vi "Initialise.vi"(8 "error in (no error)":errorcluster, 11 "Actor in":refnum<class "Status Window.lvclass">) -> (0 "error out":errorcluster, 3 "Actor out":refnum<class "Status Window.lvclass">, 5 "Observers":cluster{"Actor":refnum<event-registration>})   [LabVIEW 2015, in "Status Window.lvclass"]
uses:
  Status Window.lvclass
  Re-use Libraries/Minimal Actor Framework/Messaging/Message/Message.lvclass
  Re-use Libraries/Utility/Utility.lvlib
  Re-use Libraries/Minimal Actor Framework/Actors/Base Actor/Actor/Actor.lvclass
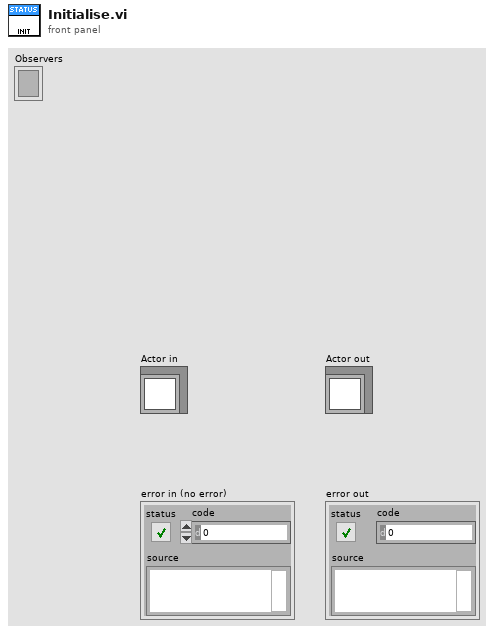
[diagram p1: front panel]
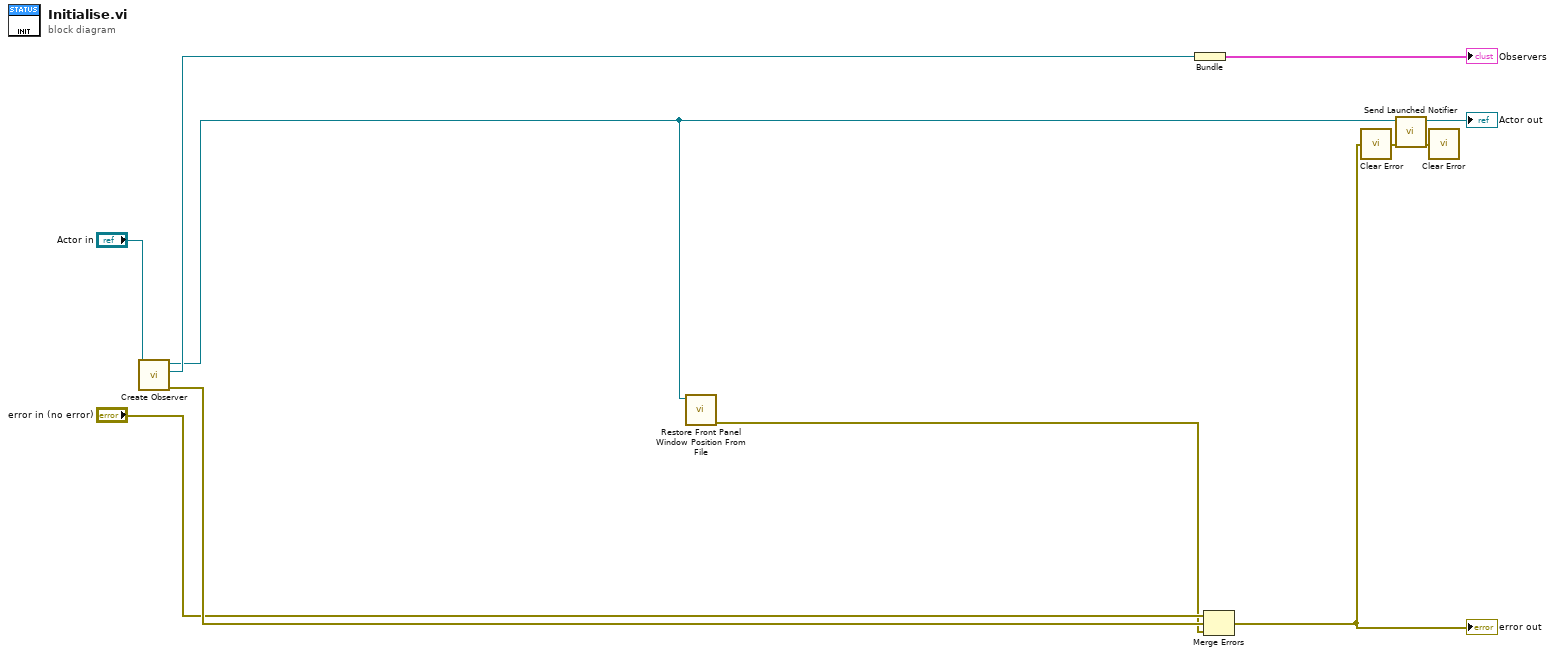
[diagram p0: block diagram]
diagram:
  n1 = call-dynamic "Create Observer.vi"("Actor in"="Actor in") -> ("error out"=w9:errorcluster, "Actor"=w4:refnum<event-registration>, "Actor out"=w1:refnum<class "Status Window.lvclass">)  [unwired: 8 in]
  n2 = call "Restore Front Panel Window Position From File.vi"("Actor in"=w1) -> ("error out"=w2:errorcluster)  [unwired: 10 in]
  n3 = Bundle("Actor"=w4) -> (→"Observers":cluster{"Actor":refnum<event-registration>})  [unwired: 1 in]
  n4 = Merge Errors("error in (no error)", w9, w2) -> (w8:errorcluster)
  "error out" <- w8
  n5 = call "Clear Error.vi"("error in (no error)"=w8) -> ("error out"=w7:errorcluster)
  n6 = call-dynamic "Send Launched Notifier.vi"("error in (no error)"=w7, "Actor in"=w1) -> ("error out"=w6:errorcluster, "Actor out"=→"Actor out":refnum<class "Status Window.lvclass">)  [unwired: 8 in]
  n7 = call "Clear Error.vi"("error in (no error)"=w6) -> ()  [unwired: 1 out]
